vi "Subsystem Sequencer Get Queue.vi"(8 "error in (no error)":errorcluster) -> (0 "error out":errorcluster, 3 "queue out":refnum<queue>)   [LabVIEW 2018]
uses:
  Sequencer Type.ctl
  All Commands.ctl
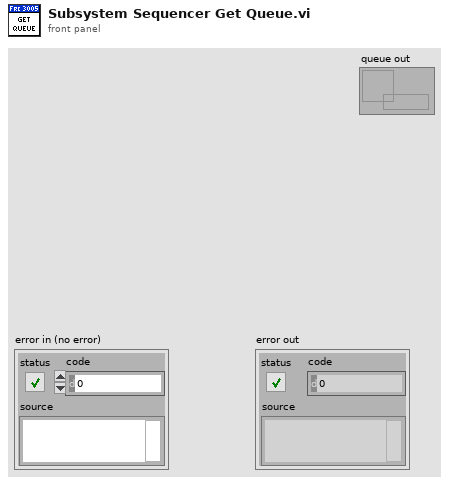
[diagram p1: front panel]
types:
  T1 = typedef "Sequencer Type.ctl" = cluster{"Cmd":T2, "Value":dbl}
  T2 = typedef "All Commands.ctl" = enum16{"Wait ms", "Drive - Stop Driving", "Drive - Drive Distance Straight", "Elevator - Elevator Stop", "Elevator - Elevator Set Position Wait", "Elevator - Elevator Set Position Start", "Elevator - Wait for Down Fast", "Wrist - Up", "Wrist - Down", "Wrist - Set Position", "Beak - Extend", "Beak - Retract", "Beak - Open", "Beak - Close", "Roller - Off", "Roller - Out", "Roller - In", "Roller - Set Position", "Roller - Wait for Cargo", "Drive - Set Power Straight", "Elevator - Wait Until Stopped", "Leg  - Piston Engage", "Wrist - Set Position Override"}
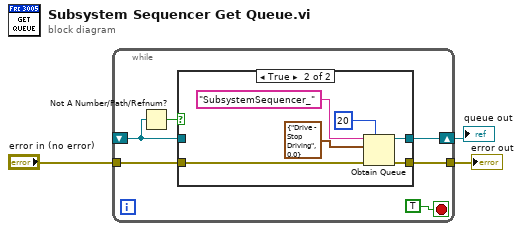
[diagram p0: block diagram]
diagram:
  n1 = while {
    shift-right: [w8] -> w1
    shift-left: _ -> [w4]
    tunnel: "error in (no error)" -> [w7]
    tunnel: [w6] -> w2
    stop <- TRUE stop-if-true
    n2 = Not A Number/Path/Refnum?(number/path/refnum=w4) -> (NaN/Path/Refnum?=w5:bool)
    n3 = case shown="True" w5 {
      tunnel: [w10 w14] -> w8
      tunnel: w7 -> [w11 w13]
      tunnel: [w11 w12] -> w6
      tunnel: w4 -> [w10 _]
      frame False {
      }
      frame True {
        n4 = Obtain Queue(max queue size (-1, unlimited)=20, name (unnamed)="SubsystemSequencer_", element data type=T1 {"Cmd"=enum."Drive - Stop Driving", "Value"=0.0}, error in (no error)=w13) -> (queue out=w14:refnum<queue>, error out=w12:errorcluster)  [unwired: 1 in, 1 out]
      }
    }
  }
  "error out" <- w2
  "queue out" <- w1
